vi "自定义单按钮对话框.vi"(9 "确定":string, 11 "消息":string) -> ()   [LabVIEW 2016, in "数据传输系统-05.lvlib"]
uses:
  <vilib>/Platform/TimedLoop/XDataNode/timing_clust.ctl
  <vilib>/Platform/TimedLoop/XDataNode/nitl_modes.ctl
  <vilib>/Platform/TimedLoop/XDataNode/wakeup.ctl
  <vilib>/Platform/TimedLoop/XDataNode/XDataNode.xnode
  <vilib>/Platform/TimedLoop/XDataNode/XDNodeRunTimeDep.lvlib
panel:
  out "计时":i32
  in  "确定":bool
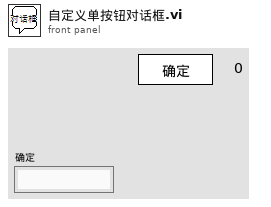
[diagram p1: front panel]
types:
  T1 = typedef "XDNodeRunTimeDep.lvlib/timing_clust.ctl" = cluster{"Expected End [f-1]":u64, "Actual End [f-1]":u64, "Finished Late? [f-1]":bool, "Expected End [i-1]":u64, "Actual End [i-1]":u64, "Finished Late? [i-1]":bool, "Expected Start [i]":u64, "Actual Start [i]":u64, "Expected Start [f]":u64, "Actual Start [f]":u64, "Source Name":string, "Structure Name":string, "Period":i64, "Deadline":i64, "Offset":i64, "Start":i64, "Priority":i32, "Timeout":i32, "Mode":T2, "Wakeup Reason":T3, "Error":errorcluster, "Source Type":string, "Secondary Source Type":string, "Global End Time":u64, "Global Start Time":u64, "Frame Duration":u64, "Iteration Duration":u64, "Assigned CPU":i32, "I/O Scan Engine Mode":u32}
  T2 = typedef "XDNodeRunTimeDep.lvlib/nitl_modes.ctl" = enum32{"No Change", "Process missed periods, maintain original phase", "Discard missed periods, maintain original phase", "Process missed periods, ignore original phase", "Discard missed periods, ignore original phase"}
  T3 = typedef "XDNodeRunTimeDep.lvlib/wakeup.ctl" = enum32{"Normal", "Aborted", "Asynchronous wakeup", "Timing source error", "Timed loop error", "Timeout"}
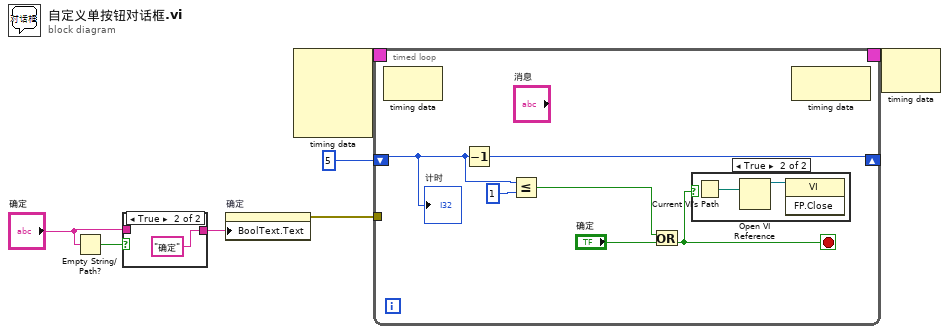
[diagram p0: block diagram]
diagram:
  n1 = Empty String/Path?(string/path="确定") -> (empty?=w3:bool)
  n2 = case shown="True" w3 {
    tunnel: [w8 "确定"] -> w2
    tunnel: "确定" -> [w8 _]
    frame False {
    }
    frame True {
    }
  }
  n3 = property on="确定" class="Bool"("BoolText.Text"=w2) -> (error out=w4:errorcluster)  [unwired: 2 in, 1 out]
  n4 = node-c288() -> (w7:T1)  [unwired: 4 in]
  n5 = timed-loop {
    timing: w7 -> [_]
    timing-out: [_] -> w6
    shift-right: [w14] -> _
    shift-left: 5 -> [w13]
    tunnel: w4 -> [_]
    stop <- w10 stop-if-true
    n6 = node-c288() -> ()  [unwired: 1 in, 1 out]
    n7 = Decrement(x=w13) -> (x-1=w14:i32)
    n8 = Less Or Equal?(x=w13, y=1) -> (x <= y?=w11:bool)
    n9 = Or(x=w11, y="确定") -> (x .or. y?=w10:bool)
    n10 = case shown="True" w10 {
      frame False {
      }
      frame True {
        n11 = Current VI's Path() -> (path=w17:path)
        n12 = Open VI Reference(vi path=w17) -> (vi reference=w16:refnum<vi>)  [unwired: 5 in, 1 out]
        n13 = invoke class="VI" method="FP.Close"(reference=w16) -> ()  [unwired: 2 in, 3 out]
      }
    }
    n14 = node-c288() -> ()  [unwired: 1 in, 1 out]
    "计时" <- w13
  }
  n15 = node-c288(w6) -> ()  [unwired: 1 out]
